vi "Dashboard Main.vi"() -> ()   [LabVIEW 2018]
uses:
  <vilib>/Utility/miscctls.llb/LVRowAndColumnTypeDef.ctl
  <vilib>/event_ctls.llb/eventvkey.ctl
  <vilib>/Rock Robotics/Network Tables/NT Read Numeric Array.vi
  <vilib>/Rock Robotics/WPI/Dashboard/WPI_DashboardLogging Global.vi
  <vilib>/vision/NI_Vision_Development_Module.lvlib
panel:
  in  "Camera Settings Right":T1={"Frame Rate"=30, "Compression"=30, "Size"=1, "DB Camera Config"=FALSE} {"Frame Rate" scale=1.0..30.0; "Compression" scale=100.0..-1.0; "Size" items=["640x480", "320x240", "160x120"]}
  in  "Camera Name Right":string(combo)="No Camera Selection"
  out "Camera Perf":string
  in  "Camera Settings":T1={"Frame Rate"=30, "Compression"=30, "Size"=1, "DB Camera Config"=FALSE} {"Frame Rate" scale=1.0..30.0; "Compression" scale=100.0..-1.0; "Size" items=["640x480", "320x240", "160x120"]}
  in  "TCP":refnum<k5>
  in  "Rec Mode":enum32{"Stop", "Record", "Playback"}(radio)
  out "Robot IP":string
  out "Image Message":string="Timeout in Camera Communications"
  in  "Dashboard Tab":T2(tab)
  in  "Select Auto":string(combo)="Select Autonomous ..."
  out "NT Connection":bool
  out "MotorChart R":cluster{"Numeric":dbl, "Numeric":dbl}(graph)
  out "MotorChart L":cluster{"Numeric":dbl, "Numeric":dbl}(graph)
  out "MotorSliders R":cluster{"MotorSlide1":dbl, "MotorSlide2":dbl} {"MotorSlide2" scale=-1.0..1.0 scale format="%#_2e"; "MotorSlide1" scale=-1.0..1.0 scale format="%#_2e"}
  out "MotorSliders L":cluster{"MotorSlide1":dbl, "MotorSlide2":dbl} {"MotorSlide2" scale=-1.0..1.0 scale format="%#_2e"; "MotorSlide1" scale=-1.0..1.0 scale format="%#_2e"}
  out "Gyro":dbl(knob) scale=0.0..360.0
  out "JS1 Z":dbl(slide) scale=-1.0..1.0 scale format="%#_2e"
  out "JS1 Graph":cluster{"X":dbl, "Y":dbl}[](graph)
  out "JS1 Buttons":T3
  out "JS2 Z":dbl(slide) scale=-1.0..1.0 scale format="%#_2e"
  out "JS2 Graph":cluster{"X":dbl, "Y":dbl}[](graph)
  out "JS2 Buttons":T3
  out "Mode":T4(ring)=enum."Auto Disabled"
  out "Right Camera Perf":cluster{"Bandwidth (Mbps)":dbl, "FPS":dbl}
  out "Camera Image Right":T5(plugin-control)
  in  "DB/String 9":string
  in  "DB/String 8":string
  in  "DB/String 7":string
  in  "DB/String 6":string
  in  "DB/String 5":string
  in  "DB/String 4":string
  in  "DB/String 3":string
  in  "DB/String 2":string
  in  "DB/String 1":string
  in  "DB/String 0":string
  in  "DB/Slider 0":dbl(slide) scale=0.0..5.0
  in  "DB/Slider 1":dbl(slide) scale=0.0..5.0
  in  "DB/Slider 2":dbl(slide) scale=0.0..5.0
  in  "DB/Slider 3":dbl(slide) scale=0.0..5.0
  out "DB/LED 3":bool
  out "DB/LED 2":bool
  out "DB/LED 1":bool
  out "DB/LED 0":bool
  in  "DB/Button 3":bool
  in  "DB/Button 2":bool
  in  "DB/Button 1":bool
  in  "DB/Button 0":bool caption="New Name"
  in  "Test Slider":dbl(slide) scale=0.0..100.0 scale format="%#_3g"
  in  "On/Off":bool caption="Solenoid"
  in  "Test Name":u16(ring) items=["Select the test to run..."]
  in  "Test Tree":string(tree)
  in  "Motor":cluster{"Value":dbl, "Enable":bool} {"Value" scale=-1.0..1.0 scale format="%#_3g"}
  out "Progress":T6 {"Test Progress" scale=0.0..100.0}
  in  "Rev/Fwd":cluster{"Forward":bool, "Reverse":bool}
  in  "Test Ring":u16(ring) items=["Monochrome", "Color"]
  out "Cmd Status":string
  in  "Execute Command":bool
  in  "Command Params":string[][](table)
  in  "Command Selection":i32(listbox)
  in  "CheckList":i32(listbox)
  out "Tree":string(tree)
  out "Camera Image":T5(plugin-control)
  out "Background":bool
  in  "Camera Name":string(combo)="No Camera Selection"
  # "HW"
  # "HW"
  # "Joysticks"
  # "Drive Motors"
  # "Front"
  # "Right"
  # "Left"
  # "Back"
  # "This tab is a great place for autonomous settings and robot-specific values.\nPlace controls and indicators inside this tab and match name to\nDashboard Variables on robot. You can also delete this comment."
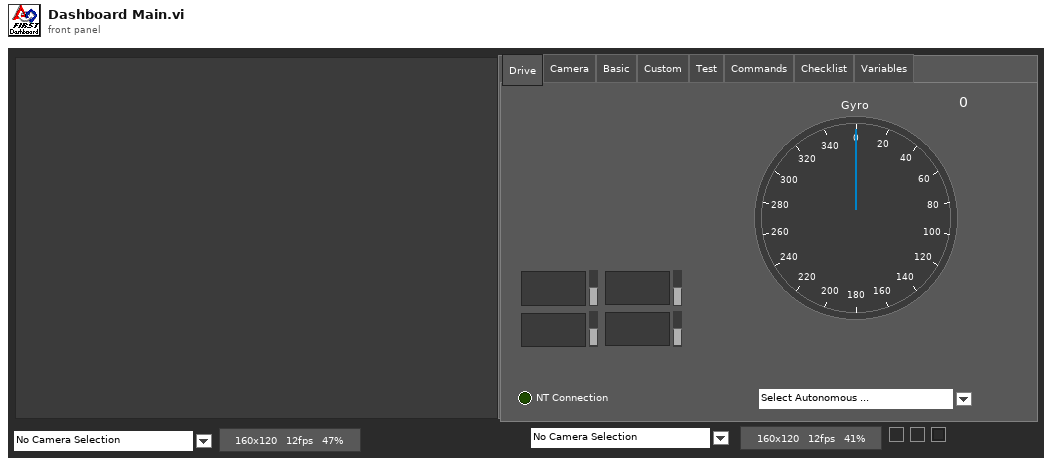
[diagram p1: front panel]
types:
  T1 = cluster{"Frame Rate":i32, "Compression":i32, "Size":u16, "DB Camera Config":bool}
  T2 = enum32{"Drive", "Camera", "Basic", "Custom", "Test", "Commands", "Checklist", "Variables"}
  T3 = cluster{bool, bool, bool, bool, bool, bool, bool, bool, bool, bool, bool, bool}
  T4 = enum8{"Tele-Op Disabled", "Tele-Op Enabled", "Auto Disabled", "Auto Enabled", "Test Disabled", "Test Enabled", "Disconnected", "No Code", "E-Stop"}
  T5 = typedef "IMAQ Image.ctl" = refnum<image>
  T6 = cluster{"Test Progress":u8, "Test Progress Text":string}
  T7 = typedef "Image Type" = u32
  T8 = cluster{"Save Path":path, "Interval (s)":dbl, "Keep":i32}
  T9 = cluster{"IDs":cluster{"RPC field ID":u16, "Unique ID":u16}, "String":string}
  T10 = cluster{"Error Strings":string, "Disable Counts":cluster{u16, u16}, "Rail Faults":cluster{u16, u16, u16}, "Robot IP":string, "DB Mode":u8, "Event Info":cluster{"Name":string, "Type":u8, "Number":u16, "Replay":u8}}
  T11 = cluster{"Storage":cluster{"Disk Free":u64, "RAM Block":u32, "RAM free":u32}, "CPU Utilization":cluster{"CPU % ISR":sgl, "CPU % Time Crit":sgl, "CPU % Timed Str":sgl, "CPU % High":sgl, "CPU % Above":sgl, "CPU % Normal":sgl, "CPU % Low":sgl}, "CAN":cluster{"% Bus Utilization":sgl, "Bus Off Cnt":u32, "TX_FIFO Full Cnt":u32, "Receive Error Cnt":u8, "Transmit Error Cnt":u8}, "HID":cluster{"HID Outputs":u32, "Rumble Low":u16, "Rumble High":u16}[]}
  T12 = cluster{"Status bits":cluster{"Test Mode":bool, "Autonomous":bool, "Enabled":bool, "Code Start":bool, "Brownout":bool, "Reserved 2":bool, "Reserved 3":bool, "E-Stop":bool}, "Code Trace":cluster{"Disabled":bool, "TeleOp":bool, "Auto":bool, "Test":bool}, "Controller Type":enum16{"unknown", "cRIO", "roboRio"}, "Code?":enum16{"unknown", "noCode", "code"}, "Battery V":dbl}
  T13 = cluster{"Control Bits":cluster{"TestMode":bool, "Autonomous":bool, "Enabled":bool, "FMS Present":bool, bool, bool, bool, "E-Stop":bool}, "Team Station ":u8, "Countdown":sgl, "Joystick Values":cluster{"Axes":dbl[], "Buttons":bool[], "POVs":i16[]}[]}
  T14 = cluster{"Axes":dbl[], "Buttons":bool[], "POVs":i16[]}[]
  T15 = cluster{"Axes":dbl[], "Buttons":bool[], "POVs":i16[]}
  T16 = cluster{"Buttons[0]":bool, "Buttons[1]":bool, "Buttons[2]":bool, "Buttons[3]":bool, "Buttons[4]":bool, "Buttons[5]":bool, "Buttons[6]":bool, "Buttons[7]":bool, "Buttons[8]":bool, "Buttons[9]":bool, "Buttons[10]":bool, "Buttons[11]":bool}
  T17 = cluster{"Camera Image":refnum<vi>, "Dashboard Tab":refnum<vi>, "Background":refnum<vi>, "Rec Mode":refnum<vi>, "Test Slider":refnum<vi>, "On/Off ":refnum<vi>, "Test Ring":refnum<vi>, "Rev/Fwd":refnum<vi>, "Test Name":refnum<vi>, "Motor":refnum<vi>, "Progress":refnum<vi>, "CheckList":refnum<vi>, "Tree":refnum<vi>, "Test Tree":refnum<vi>, "Command Params":refnum<vi>, "Command Selection":refnum<vi>, "Execute Command":refnum<vi>, "Cmd Status":refnum<vi>, "Camera Settings":refnum<vi>, "Camera Name":refnum<vi>, "Camera Perf":refnum<vi>, "Camera Settings Right":refnum<vi>, "Camera Name Right":refnum<vi>, "Camera Image Right":refnum<vi>}
  T18 = cluster{"Global Rectangle":i32[], "Contours":cluster{"Contour Type":u32, "ROI Type":u32, "Points":i32[]}[]}
  T19 = cluster{"Camera Name":string, string, "Saved DB Images Info":cluster{"Save Path":path, "Interval (s)":dbl, "Keep":i32}}
  T20 = cluster{"Camera Name Right":string, string, "Saved DB Images Info":cluster{"Save Path":path, "Interval (s)":dbl, "Keep":i32}}
  T21 = cluster{"Operation":enum16{"Update", "Clear"}, "Color Box":u32}[]
  T22 = typedef "eventvkey.ctl" = enum16{"ASCII", "Enter", "Return", "Shift", "Ctrl", "Alt", "Cmd", "Opt", "Caps", "NumLock", "Clear", "Break", "Up", "Down", "Left", "Right", "Insert", "Delete", "Home", "End", "PageUp", "PageDown", "Escape", "Help", "Pause", "ScrollLock", "F1", "F2", "F3", "F4", "F5", "F6", "F7", "F8", "F9", "F10", "F11", "F12", "F13", "F14", "F15", "F16", "F17", "F18", "F19", "F20", "F21", "F22", "F23", "F24", "Play", "VolumeUp", "VolumeDown", "Mute", "Two Byte Char"}
  T23 = cluster{"Image Size":bool, "Image Type":bool, "Pixel Value":bool, "ROI Information":bool, "Zoom Factor":bool}
  T24 = cluster{"Operation":enum16{"Update", "Clear"}, "Color Box":u32}
  T25 = typedef "LVRowAndColumnTypeDef.ctl" = cluster{"Row":i32, "Column":i32}
  T26 = cluster{"Shift":bool, "Ctrl":bool, "Alt":bool, "Cmd":bool, "Opt":bool}
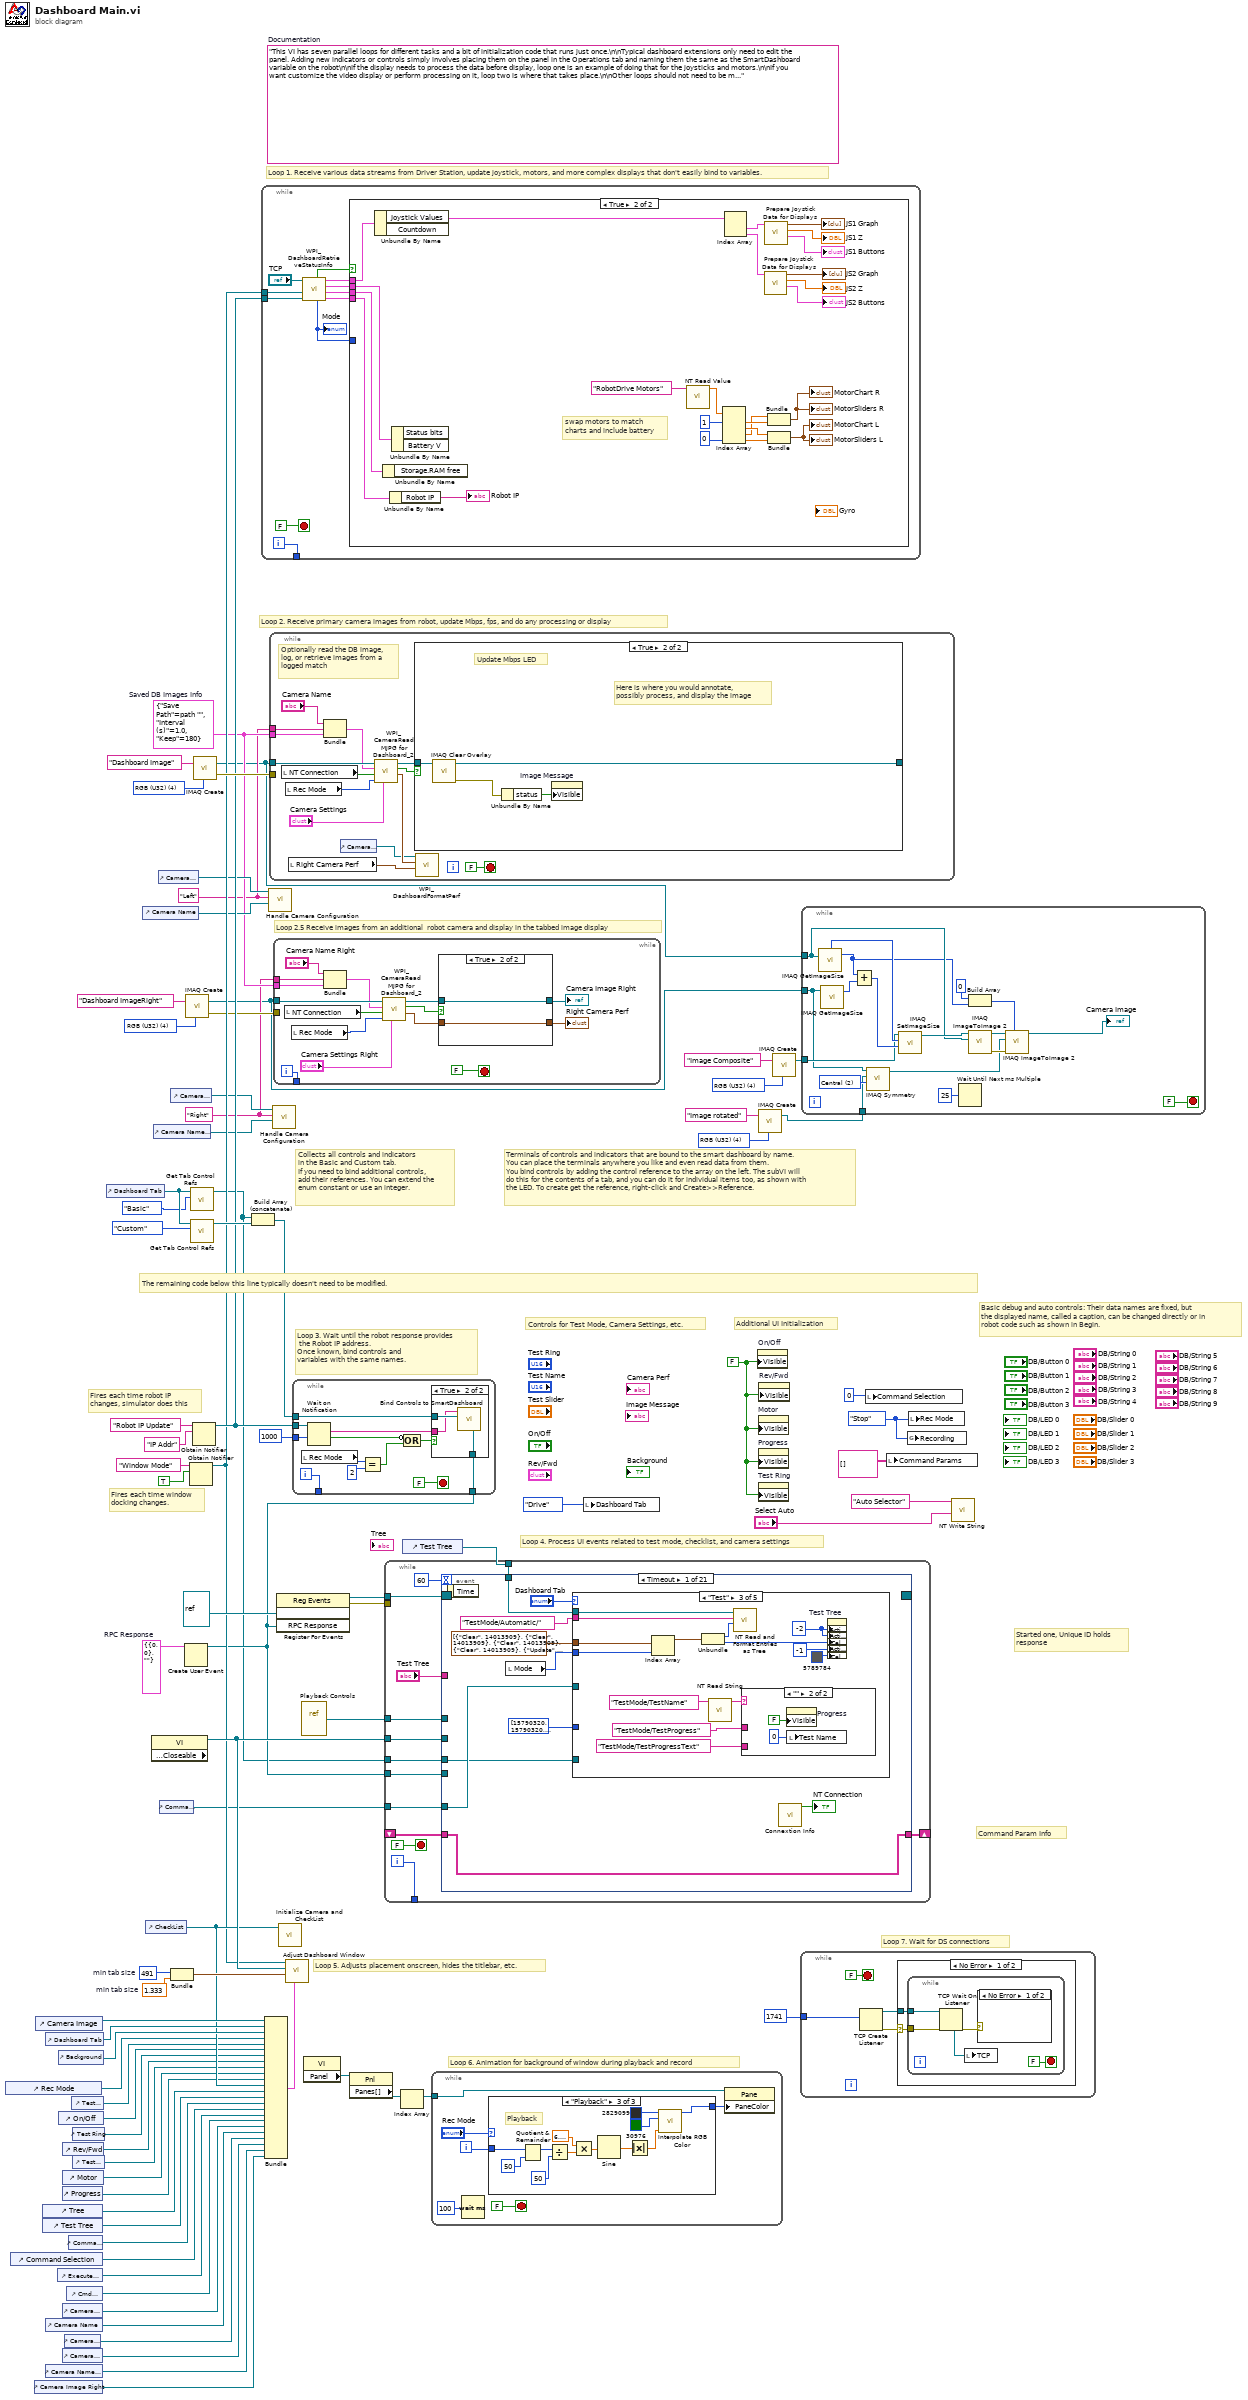
[diagram p0: block diagram]
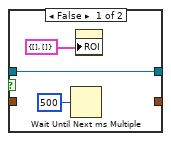
[diagram p2: hidden frame]
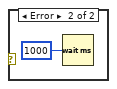
[diagram p3: hidden frame]
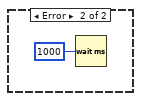
[diagram p4: hidden frame]
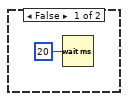
[diagram p5: hidden frame]
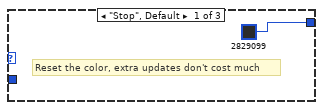
[diagram p6: hidden frame]
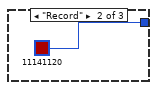
[diagram p7: hidden frame]
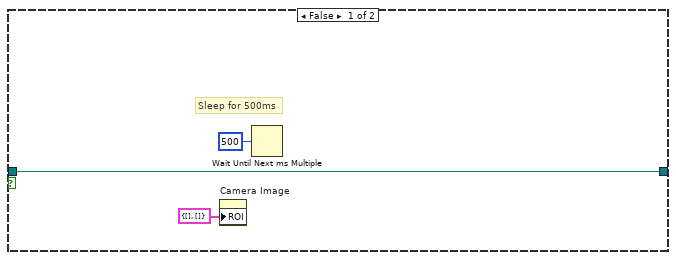
[diagram p9: hidden frame]
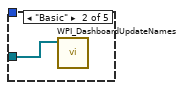
[diagram p11: hidden frame]
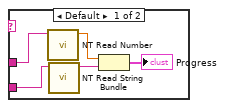
[diagram p12: hidden frame]
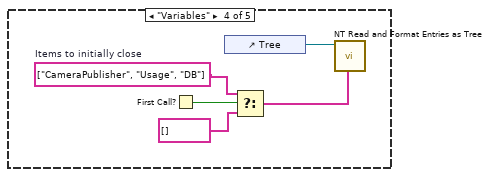
[diagram p13: hidden frame]
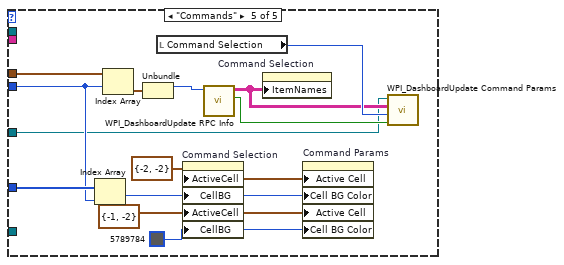
[diagram p14: hidden frame]
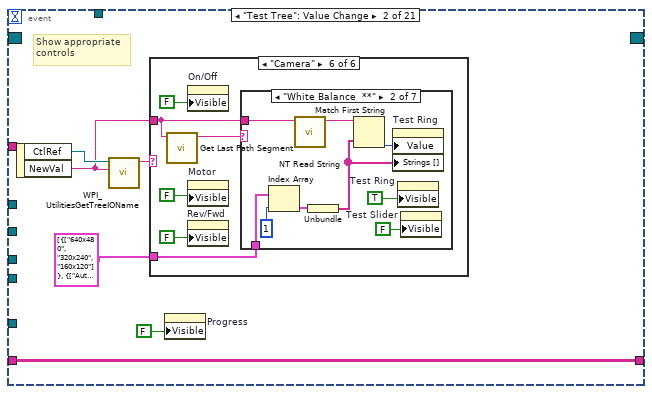
[diagram p15: hidden frame]
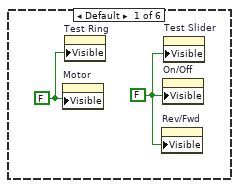
[diagram p16: hidden frame]
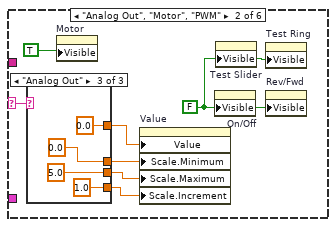
[diagram p17: hidden frame]
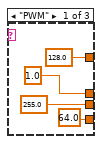
[diagram p18: hidden frame]
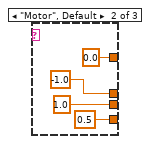
[diagram p19: hidden frame]
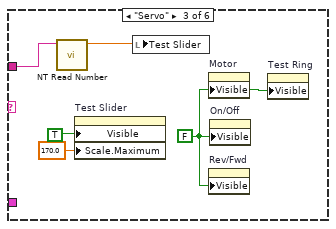
[diagram p20: hidden frame]
diagram:
  w2 = T7 4 items=["Grayscale (U8)", "Grayscale (I16)", "Grayscale (SGL)", "Complex (CSG)", "RGB (U32)", "HSL (U32)", "RGB (U64)"] ("Image Type")
  w8 = T7 4 items=["Grayscale (U8)", "Grayscale (I16)", "Grayscale (SGL)", "Complex (CSG)", "RGB (U32)", "HSL (U32)", "RGB (U64)"] ("Image Type")
  w11 = T8 {"Save Path"=path "", "Interval (s)"=1.0, "Keep"=180}  # Saved DB Images Info
  w10 = "Right"
  w9 = "Left"
  w20 = T7 4 items=["Grayscale (U8)", "Grayscale (I16)", "Grayscale (SGL)", "Complex (CSG)", "RGB (U32)", "HSL (U32)", "RGB (U64)"] ("Image Type")
  w36 = T9 {"IDs"={"RPC field ID"=0, "Unique ID"=0}, "String"=""}  # RPC Response
  w59 = 491  # min tab size
  w58 = 1.333  # min tab size
  w66 = enum32{"Stop", "Record", "Playback"}."Stop" ("Rec Mode")
  w43 = FALSE ("Visible")
  (unwired) "This VI has seven parallel loops for different tasks and a bit of initialization code that runs just once.\n\nTypical dashboard extensions only need to edit the panel. Adding new indicators or controls simply involves placing them on the panel in the Operations tab and naming them the same as the SmartDashboard variable on the robot\n\nIf the display needs to process the data before display, loop one is an example of doing that for the joysticks and motors.\n\nIf you want customize the video display or perform processing on it, loop two is where that takes place.\n\nOther loops should not need to be modified. They are pretty standard, and document the task they perform."  # Documentation
  w82 = T7 4 items=["Grayscale (U8)", "Grayscale (I16)", "Grayscale (SGL)", "Complex (CSG)", "RGB (U32)", "HSL (U32)", "RGB (U64)"] ("Image Type")
  # "Loop 2.5 Receive images from an additional  robot camera and display in the tabbed image display"
  # "Command Param Info"
  # "Started one, Unique ID holds\nresponse"
  # "Loop 7. Wait for DS connections"
  # "Basic debug and auto controls: Their data names are fixed, but\nthe displayed name, called a caption, can be changed directly or in\nrobot code such as shown in Begin."
  # "Controls for Test Mode, Camera Settings, etc."
  # "Additional UI Initialization"
  # "Loop 6. Animation for background of window during playback and record"
  # "Fires each time robot IP\nchanges, simulator does this"
  # "Fires each time window\ndocking changes."
  # "Collects all controls and indicators\nin the Basic and Custom tab.\nIf you need to bind additional controls,\nadd their references. You can extend the\nenum constant or use an integer."
  # "The remaining code below this line typically doesn't need to be modified."
  # "Loop 4. Process UI events related to test mode, checklist, and camera settings"
  # "Terminals of controls and indicators that are bound to the smart dashboard by name.\nYou can place the terminals anywhere you like and even read data from them.\nYou bind controls by adding the control reference to the array on the left. The subVI will\ndo this for the contents of a tab, and you can do it for individual items too, as shown with\nthe LED. To create get the reference, right-click and Create>>Reference."
  # "Loop 3. Wait until the robot response provides\n the Robot IP address.\nOnce known, bind controls and\nvariables with the same names."
  # "Loop 5. Adjusts placement onscreen, hides the titlebar, etc."
  # "Loop 1. Receive various data streams from Driver Station, update joystick, motors, and more complex displays that don't easily bind to variables."
  # "Loop 2. Receive primary camera images from robot, update Mbps, fps, and do any processing or display"
  n1 = control-ref of="Rec Mode"() -> (w49:refnum<vi>)
  n2 = control-ref of="Command Selection"() -> (w35:refnum<vi>)
  n3 = control-ref of="Camera Image Right"() -> (w14:refnum<vi>)
  n4 = control-ref of="Camera Image"() -> (w61:refnum<vi>)
  n5 = control-ref of="Tree"() -> (w53:refnum<vi>)
  n6 = control-ref of="Test Tree"() -> (w52:refnum<vi>)
  n7 = control-ref of="Dashboard Tab"() -> (w60:refnum<vi>)
  n8 = control-ref of="Camera Name"() -> (w26:refnum<vi>)
  n9 = control-ref of="Camera Name Right"() -> (w15:refnum<vi>)
  n10 = control-ref of="Execute Command"() -> (w37:refnum<vi>)
  n11 = control-ref of="Background"() -> (w56:refnum<vi>)
  n12 = control-ref of="On/Off"() -> (w47:refnum<vi>)
  n13 = control-ref of="Progress"() -> (w44:refnum<vi>)
  n14 = control-ref of="Camera Settings"() -> (w27:refnum<vi>)
  n15 = control-ref of="Camera Settings Right"() -> (w16:refnum<vi>)
  n16 = control-ref of="Rev/Fwd"() -> (w45:refnum<vi>)
  n17 = control-ref of="Motor"() -> (w50:refnum<vi>)
  n18 = control-ref of="Camera Perf"() -> (w25:refnum<vi>)
  n19 = control-ref of="Cmd Status"() -> (w31:refnum<vi>)
  n20 = control-ref of="Command Params"() -> (w38:refnum<vi>)
  n21 = control-ref of="Test Slider"() -> (w48:refnum<vi>)
  n22 = control-ref of="Test Ring"() -> (w46:refnum<vi>)
  n23 = control-ref of="Test Name"() -> (w51:refnum<vi>)
  n24 = control-ref of="Dashboard Tab"() -> (w64:refnum<vi>)
  n25 = control-ref of="Camera Name"() -> (w28:refnum<vi>)
  n26 = control-ref of="CheckList"() -> (w54:refnum<vi>)
  n27 = property class="VI" props=["Front Panel.Closeable"]() -> (reference out=w65:refnum<vi>)  [unwired: 2 in, 2 out]
  n28 = control-ref of="Camera Name Right"() -> (w17:refnum<vi>)
  n29 = control-ref of="Camera Settings"() -> (w29:refnum<vi>)
  n30 = control-ref of="Command Params"() -> (w30:refnum<vi>)
  n31 = control-ref of="Camera Settings Right"() -> (w18:refnum<vi>)
  n32 = Bundle("min tab size"=w59, "min tab size"=w58) -> (w57:cluster{"min tab size":i32, "min tab size":dbl})  [unwired: 1 in]
  n33 = Create User Event(user event datatype=w36) -> (user event=w32:refnum<user-event>)  [unwired: 1 in, 1 out]
  n34 = call "IMAQ Create"("Image Name"="Dashboard ImageRight", "Image Type"=w20) -> ("New Image"=w5:T5, "error out"=w19:errorcluster)  [unwired: 2 in, 1 out]
  n35 = Obtain Notifier(name (unnamed)="Window Mode", notification data type=TRUE) -> (notifier out=w41:refnum<notifier>)  [unwired: 2 in, 2 out]
  n36 = call <vilib>:"Get Tab Control Refs.vi"("Page Index"=T2."Basic" ("Dashboard Tab"), "TabControl in"=w64) -> ("ControlsOnPage"=w24:refnum<vi>[])  [unwired: 9 in]
  n37 = call <vilib>:"Get Tab Control Refs.vi"("Page Index"=T2."Custom" ("Dashboard Tab"), "TabControl in"=w64) -> ("ControlsOnPage"=w63:refnum<vi>[])  [unwired: 9 in]
  n38 = Obtain Notifier(name (unnamed)="Robot IP Update", notification data type="IP Addr" ("name (unnamed)")) -> (notifier out=w42:refnum<notifier>)  [unwired: 2 in, 2 out]
  n39 = call "IMAQ Create"("Image Name"="Dashboard Image", "Image Type"=w82) -> ("New Image"=w6:T5, "error out"=w80:errorcluster)  [unwired: 2 in, 1 out]
  n40 = Build Array (concatenate)(w24, w63) -> (w62:refnum<vi>[])
  n41 = while {
    tunnel: [w92] -> _
    tunnel: w42 -> [w86]
    tunnel: w41 -> [w83]
    i -> [w92]
    stop <- FALSE stop-if-true
    n42 = call <vilib>:"WPI_DashboardRetrieveStatusInfo.vi"("Binding Refnum"=w86, "Window Mode Notifier"=w83, "TCP Cnx"="TCP") -> ("Power and Errors"=w87:T10, "Robot Metrics"=w90:T11, "Status Info"=w91:T12, "Control Info"=w88:T13, "Robot Mode"=w85:T4, "Process?"=w89:bool)  [unwired: 3 in]
    "Mode" <- w85
    n43 = case shown="True" w89 {
      tunnel: w91 -> [_ w118]
      tunnel: w90 -> [_ w117]
      tunnel: w88 -> [_ w116]
      tunnel: w87 -> [_ w115]
      tunnel: w85 -> [_ _]
      frame False {
        n44 = Wait (ms)(milliseconds to wait=u32 20) -> ()  [unwired: 1 out]
      }
      frame True {
        # "swap motors to match\ncharts and include battery"
        n45 = Unbundle By Name(w116) -> ("Joystick Values"=w106:T14)  [unwired: 1 out]
        n46 = Unbundle By Name(w117) -> ()  [unwired: 1 out]
        n47 = Unbundle By Name(w115) -> ("Robot IP"=→"Robot IP":string)
        n48 = Unbundle By Name(w118) -> ()  [unwired: 2 out]
        n49 = call-poly <vilib>:"NT Read Value.vi"("Name"="RobotDrive Motors") -> ("Numeric Array"=w96:dbl[])  [unwired: 9 in, 1 out]
        n50 = Index Array(array=w96, index #1=1, index #4=0) -> (element #1=w110:dbl, element #2=w111:dbl, element #3=w109:dbl, element #4=w114:dbl)  [unwired: 2 in]
        n51 = Index Array(array=w106) -> (element #1=w105:T15, element #2=w101:T15)  [unwired: 2 in]
        n52 = call "Prepare Joystick Data for Displays.vi"("Joystick Values"=w101) -> ("Buttons"=→"JS2 Buttons":T16, "Z Axis"=→"JS2 Z":dbl, "Cartesian Data"=→"JS2 Graph":cluster{"X axis":dbl, "X axis":dbl}[])  [unwired: 8 in]
        n53 = call "Prepare Joystick Data for Displays.vi"("Joystick Values"=w105) -> ("Buttons"=→"JS1 Buttons":T16, "Z Axis"=→"JS1 Z":dbl, "Cartesian Data"=→"JS1 Graph":cluster{"X axis":dbl, "X axis":dbl}[])  [unwired: 8 in]
        n54 = Bundle("Numeric"=w109, "Numeric"=w110) -> (→"MotorChart R" →"MotorSliders R":cluster{"Numeric":dbl, "Numeric":dbl})  [unwired: 1 in]
        n55 = Bundle("Numeric"=w111, "Numeric"=w114) -> (→"MotorChart L" →"MotorSliders L":cluster{"Numeric":dbl, "Numeric":dbl})  [unwired: 1 in]
      }
    }
  }
  n56 = Bundle("Camera Image"=w61, "Dashboard Tab"=w60, "Background"=w56, "Rec Mode"=w49, "Test Slider"=w48, "On/Off"=w47, "Test Ring"=w46, "Rev/Fwd"=w45, "Test Name"=w51, "Motor"=w50, "Progress"=w44, "CheckList"=w54, "Tree"=w53, "Test Tree"=w52, "Command Params"=w38, "Command Selection"=w35, "Execute Command"=w37, "Cmd Status"=w31, "Camera Settings"=w27, "Camera Name"=w26, "Camera Perf"=w25, "Camera Settings Right"=w16, "Camera Name Right"=w15, "Camera Image Right"=w14) -> (w55:T17)  [unwired: 1 in]
  n57 = call "Handle Camera Configuration.vi"("CameraNameRef"=w28, "Display Name"=w9, "ClusterRef"=w29) -> ()  [unwired: 9 in]
  n58 = while {
    tunnel: w6 -> [w131]
    tunnel: w80 -> [_]
    tunnel: w11 -> [w125]
    tunnel: w9 -> [w122]
    stop <- FALSE stop-if-true
    # "Optionally read the DB image,\nlog, or retrieve images from a\nlogged match"
    n59 = local read "NT Connection"() -> (w126:bool)
    n60 = local read "Rec Mode"() -> (w128:enum32{"Stop", "Record", "Playback"})
    n61 = local read "Right Camera Perf"() -> (w120:cluster{"Bandwidth (Mbps)":dbl, "FPS":dbl})
    n62 = Bundle("Camera Name"="Camera Name", w122, "Saved DB Images Info"=w125) -> (w124:T19)  [unwired: 1 in]
    n63 = control-ref of="Camera Perf"() -> (w119:refnum<vi>)
    n64 = call <vilib>:"WPI_CameraRead MJPG for Dashboard_2.vi"("Camera Settings"="Camera Settings", "Rec Mode"=w128, "NT Connection"=w126, "Capture Info"=w124, "Image in"=w131) -> ("perf info"=w121:cluster{"Bandwidth (Mbps)":dbl, "fps":dbl}, "Active"=w129:bool, "Image\\ out"=w130:T5)  [unwired: 4 in]
    n65 = case shown="True" w129 {
      tunnel: w130 -> [w134 w137]
      tunnel: [w134 w136] -> _
      frame False {
        # "Sleep for 500ms"
        n66 = property on="Camera Image" class="ImageControl"("ROI"=T18 {"Global Rectangle"=[], "Contours"=[]}) -> ()  [unwired: 2 in, 2 out]
        n67 = Wait Until Next ms Multiple(millisecond multiple=u32 500) -> ()  [unwired: 1 out]
      }
      frame True {
        # "Here is where you would annotate,\npossibly process, and display the image"
        # "Update Mbps LED"
        n68 = call "IMAQ Clear Overlay"("Image"=w137) -> ("error out"=w138:errorcluster, "Image Out"=w136:T5)  [unwired: 2 in, 7 out]
        n69 = Unbundle By Name(w138) -> ("status"=w139:bool)
        n70 = property on="Image Message" class="Str"("Visible"=w139) -> ()  [unwired: 2 in, 2 out]
      }
    }
    n71 = call <vilib>:"WPI_DashboardFormatPerf.vi"("Right Camera Perf"=w120, "Performance"=w121, "String in"=w119) -> ()  [unwired: 9 in]
  }
  n72 = call "Handle Camera Configuration.vi"("CameraNameRef"=w17, "Display Name"=w10, "ClusterRef"=w18) -> ()  [unwired: 9 in]
  n73 = while {
    tunnel: w5 -> [w154]
    tunnel: w19 -> [_]
    tunnel: [w149] -> _
    tunnel: w11 -> [w145]
    tunnel: w10 -> [w142]
    i -> [w149]
    stop <- FALSE stop-if-true
    n74 = local read "NT Connection"() -> (w146:bool)
    n75 = local read "Rec Mode"() -> (w153:enum32{"Stop", "Record", "Playback"})
    n76 = Bundle("Camera Name Right"="Camera Name Right", w142, "Saved DB Images Info"=w145) -> (w144:T20)  [unwired: 1 in]
    n77 = call <vilib>:"WPI_CameraRead MJPG for Dashboard_2.vi"("Camera Settings"="Camera Settings Right", "Rec Mode"=w153, "NT Connection"=w146, "Capture Info"=w144, "Image in"=w154) -> ("perf info"=w140:cluster{"Bandwidth (Mbps)":dbl, "fps":dbl}, "Active"=w148:bool, "Image\\ out"=w151:T5)  [unwired: 4 in]
    n78 = case shown="True" w148 {
      tunnel: w151 -> [w156 w159]
      tunnel: [w156 w159] -> w147
      tunnel: [_ w158] -> w141
      tunnel: w140 -> [_ w158]
      frame False {
        n79 = Wait Until Next ms Multiple(millisecond multiple=u32 500) -> ()  [unwired: 1 out]
        n80 = property on="Camera Image Right" class="ImageControl"("ROI"=T18 {"Global Rectangle"=[], "Contours"=[]}) -> ()  [unwired: 2 in, 2 out]
      }
      frame True {
      }
    }
    "Camera Image Right" <- w147
    "Right Camera Perf" <- w141
  }
  n81 = register-events(refnum<vi> refnum, w32) -> (reference out=w70:refnum<event-registration>, error out=w69:errorcluster)  [unwired: 2 in]
  n82 = call "Initialize Camera and CheckList.vi"("ListBox in"=w54) -> ()  [unwired: 11 in]
  n83 = call "Adjust Dashboard Window.vi"("Sizing Refnums"=w55, "Size Constraints"=w57, "VI"=w65, "WIn Mode"=w41) -> ()  [unwired: 8 in]
  n84 = while {
    tunnel: w62 -> [w171]
    tunnel: w42 -> [w169]
    tunnel: [w167] -> _
    tunnel: u32 1000 ("milliseconds to wait") -> [w166]
    tunnel: w32 -> [w160]
    i -> [w167]
    stop <- FALSE stop-if-true
    n85 = local read "Rec Mode"() -> (w162:enum32{"Stop", "Record", "Playback"})
    n86 = Wait on Notification(notifier=w169, timeout in ms (-1)=w166) -> (notification=w168:string, timed out?=w164:bool)  [unwired: 2 in, 2 out]
    n87 = Equal?(x=w162, y=u16 2 ("Rec Mode")) -> (x = y?=w163:bool)
    n88 = Compound Arithmetic op=OR(invert w164, w163) -> (w165:bool)
    n89 = case shown="True" w165 {
      tunnel: w171 -> [_ w174]
      tunnel: w168 -> [_ w173]
      tunnel: w160 -> [_ w172]
      frame False {
      }
      frame True {
        n90 = call <vilib>:"Bind Controls to SmartDashboard.vi"("RPC ref"=w172, "Bound Control Refs"=w174, "Server IP Address"=w173) -> ()  [unwired: 9 in]
      }
    }
  }
  n91 = vi-ref "Playback Controls.vi"() -> (w71:refnum<vi>)
  n92 = property class="VI"() -> ("Panel"=w73:refnum<vi>)  [unwired: 2 in, 2 out]
  n93 = property class="Pnl"(reference=w73) -> ("Panes[]"=w74:refnum<vi>[])  [unwired: 1 in, 2 out]
  n94 = Index Array(array=w74) -> (element=w72:refnum<vi>)  [unwired: 1 in]
  n95 = control-ref of="Test Tree"() -> (w75:refnum<vi>)
  n96 = while {
    tunnel: [w184] -> _
    tunnel: w75 -> [w183]
    tunnel: w71 -> [w182]
    tunnel: w70 -> [w181]
    tunnel: w69 -> [_]
    tunnel: w65 -> [w180]
    tunnel: w32 -> [w179]
    tunnel: w30 -> [w178]
    shift-right: [w177] -> _
    shift-left: _ -> [w176]
    tunnel: w24 -> [w175]
    i -> [w184]
    stop <- FALSE stop-if-true
    n97 = event shown="[0] Timeout" {
      selector: w181 -> [_ _ _ _ _ _ _ _ _ _ _ _ _ _ _ _ _ _ _ _ _]
      dyn-events: [_ _ _ _ _ _ _ _ _ _ _ _ _ _ _ _ w444 _ _ _ _] -> _
      timeout: u32 60 ("milliseconds to wait") -> [_ _ _ _ _ _ _ _ _ _ _ _ _ _ _ _ _ _ _ _ _]
      tunnel: w183 -> [w196 _ _ _ _ _ _ _ _ _ _ _ _ _ _ _ _ _ _ _ _]
      tunnel: "Test Tree" -> [_ _ _ _ _ _ _ _ _ _ _ w411 w419 w421 w425 w433 _ _ _ _ _]
      tunnel: w182 -> [_ _ _ _ _ _ _ _ _ _ _ _ _ _ _ _ w446 _ w464 _ _]
      tunnel: w180 -> [_ _ _ _ _ _ _ _ _ _ _ _ _ _ _ _ w442 _ _ _ _]
      tunnel: w179 -> [_ _ _ _ _ _ _ _ _ _ _ _ _ _ _ _ w440 _ _ _ _]
      tunnel: w178 -> [w191 _ _ _ _ _ w362 _ _ _ _ _ _ _ _ _ _ _ _ _ _]
      tunnel: [w190 w239 w341 w346 w355 w359 w360 w369 w379 w386 w398 w410 w417 w420 w424 w432 w439 w459 w461 w465 w478] -> w177
      tunnel: w176 -> [w190 w239 w341 w346 w355 w359 w360 _ _ w386 w398 w410 w417 w420 w424 w432 w439 w459 w461 w465 w478]
      tunnel: w175 -> [w188 _ _ _ _ _ _ _ _ _ _ _ _ _ _ _ _ _ _ _ _]
      event Timeout {
        n98 = event-data() -> ()  [unwired: 1 in, 1 out]
        n99 = local read "Mode"() -> (w193:T4)
        n100 = case shown="\"Test\"" "Dashboard Tab" {
          tunnel: w196 -> [_ _ w212 _ _]
          tunnel: "TestMode/Automatic/" ("Name Pattern") -> [_ _ w211 _ _]
          tunnel: T21 [{"Operation"=enum."Clear", "Color Box"=14013909}, {"Operation"=enum."Clear", "Color Box"=14013909}, {"Operation"=enum."Clear", "Color Box"=14013909}, {"Operation"=enum."Clear", "Color Box"=14013909}, {"Operation"=enum."Update", "Color Box"=14013909}, {"Operation"=enum."Update", "Color Box"=16777215}, {"Operation"=enum."Clear", "Color Box"=14013909}, {"Operation"=enum."Clear", "Color Box"=14013909}, {"Operation"=enum."Clear", "Color Box"=14013909}] -> [_ _ w204 _ w232]
          tunnel: w193 -> [_ _ w203 _ w231]
          tunnel: u32[] [15790320, 15790320, 15790320, 15790320, 16777215, 16777215, 15790320, 15790320, 15790320] -> [_ _ _ _ w237]
          tunnel: w191 -> [_ _ _ _ w225]
          tunnel: w188 -> [_ w198 _ _ _]
          frame "Custom", Default {
          }
          frame "Basic" {
            n101 = call <vilib>:"WPI_DashboardUpdateNames.vi"("Controls on Tab"=w198) -> ()  [unwired: 11 in]
          }
          frame "Test" {
            w210 = -2 ("Active Item:Row Number")
            n102 = Index Array(array=w204, index=w203) -> (element=w205:T24)
            n103 = Unbundle(w205) -> ("Operation"=w206:enum16{"Update", "Clear"}, "Color Box"=w207:u32)
            n104 = call <vilib>:"NT Read String.vi"("Name"="TestMode/TestName") -> ("String"=w201:string)  [unwired: 9 in, 1 out]
            n105 = call <vilib>:"NT Read and Format Entries as Tree.vi"("Operation"=w206, "Name Pattern"=w211, "Tree Refnum"=w212) -> ()  [unwired: 7 in, 2 out]
            n106 = case shown="\"\"" w201 {
              tunnel: "TestMode/TestProgress" ("Name") -> [w214 _]
              tunnel: "TestMode/TestProgressText" ("Name") -> [w213 _]
              frame Default {
                n107 = call <vilib>:"NT Read Number.vi"("Name"=w214) -> ("Numeric"=w215:dbl)  [unwired: 9 in, 1 out]
                n108 = call <vilib>:"NT Read String.vi"("Name"=w213) -> ("String"=w216:string)  [unwired: 9 in, 1 out]
                n109 = Bundle("Numeric"=w215, "String"=w216) -> (→"Progress":cluster{"Numeric":dbl, "String":string})  [unwired: 1 in]
              }
              frame "" {
                n110 = property on="Progress" class="Clust (strict)"("Visible"=FALSE) -> ()  [unwired: 2 in, 2 out]
                n111 = local write "Test Name"(u16 0) -> ()
              }
            }
            n112 = property on="Test Tree" class="Tree (strict)"("Active Item Row Number"=w210, "ActiveColNum"=w210, "CellBG"=w207, "Active Item Row Number"=-1 ("Active Item:Row Number"), "CellBG"=u32 5789784 ("Color Box")) -> ()  [unwired: 2 in, 2 out]
          }
          frame "Variables" {
            w222 = string[] ["CameraPublisher", "Usage", "DB"]  # Items to initially close
            n113 = First Call?() -> (First Call?: T/F=w223:bool)
            n114 = control-ref of="Tree"() -> (w224:refnum<vi>)
            n115 = Select(t=w222, s=w223, f=string[] []) -> (s? t:f=w220:string[])
            n116 = call <vilib>:"NT Read and Format Entries as Tree.vi"("Tags to  Close"=w220, "Tree Refnum"=w224) -> ()  [unwired: 8 in, 2 out]
          }
          frame "Commands" {
            w233 = u32 5789784 ("Color Box")
            w234 = T25 {"Row"=-1, "Column"=-2} ("Active Cell:Active Cell")
            w236 = T25 {"Row"=-2, "Column"=-2} ("Active Cell:Active Cell")
            n117 = Index Array(array=w237, index=w231) -> (element=w235:u32)
            n118 = Index Array(array=w232, index=w231) -> (element=w230:T24)
            n119 = Unbundle(w230) -> ("Operation"=w229:enum16{"Update", "Clear"})  [unwired: 1 out]
            n120 = local read "Command Selection"() -> (w228:i32)
            n121 = property on="Command Selection" class="MCListbox (strict)"("ActiveCell"=w236, "CellBG"=w235, "ActiveCell"=w234, "CellBG"=w233) -> ()  [unwired: 2 in, 2 out]
            n122 = call <vilib>:"WPI_DashboardUpdate RPC Info.vi"("Operation"=w229) -> ("update"=w227:bool, "commands"=w226:string[][])  [unwired: 9 in]
            n123 = property on="Command Selection" class="MCListbox (strict)"("ItemNames"=w226) -> ()  [unwired: 2 in, 2 out]
            n124 = property on="Command Params" class="Tbl (strict)"("Active Cell"=w236, "Cell BG Color"=w235, "Active Cell"=w234, "Cell BG Color"=w233) -> ()  [unwired: 2 in, 2 out]
            n125 = call <vilib>:"WPI_DashboardUpdate Command Params.vi"("Update"=w227, "NewVal"=w228, "Commands"=w226, "Param Tbl"=w225) -> ()  [unwired: 7 in, 1 out]
          }
        }
        n126 = call <vilib>:"Connextion Info.vi"() -> ("Connected"=→"NT Connection":bool)  [unwired: 10 in, 1 out]
      }
      event "Test Tree": Value Change {
        # "Show appropriate\ncontrols"
        n127 = event-data() -> ("CtlRef"=w242:refnum<vi>, "NewVal"=w240:string)  [unwired: 1 in]
        n128 = call <vilib>:"WPI_UtilitiesGetTreeIOName.vi"("NewVal"=w240, "TreeControl in"=w242) -> ("I/O Name"=w243:string)  [unwired: 9 in]
        n129 = case shown="\"Camera\"" w243 {
          selector: w243 -> [_ w250 _ w272 w281 _]
          tunnel: w240 -> [_ _ w269 w271 _ w288]
          tunnel: cluster{string[]}[] [{["640x480", "320x240", "160x120"]}, {["Auto", "Fixed indoor", "Fixed outdoor 1", "Fixed outdoor 2", "Fixed fluorescent 1", "Fixed fluorescent 2", "Hold current"]}, {["Auto", "Flicker-free 50 Hz", "Flicker-free 60 Hz", "Hold current"]}, {["None", "Prioritize frame rate", "Prioritize image quality"]}, {["Monochrome", "Color"]}] -> [_ _ _ _ _ w287]
          frame Default {
            w245 = FALSE ("Visible")
            w244 = FALSE ("Visible")
            n130 = property on="Motor" class="Clust (strict)"("Visible"=w244) -> ()  [unwired: 2 in, 2 out]
            n131 = property on="Test Ring" class="Ring (strict)"("Visible"=w244) -> ()  [unwired: 2 in, 2 out]
            n132 = property on="Rev/Fwd" class="Clust (strict)"("Visible"=w245) -> ()  [unwired: 2 in, 2 out]
            n133 = property on="On/Off" class="Bool (strict)"("Visible"=w245) -> ()  [unwired: 2 in, 2 out]
            n134 = property on="Test Slider" class="Slide (strict)"("Visible"=w245) -> ()  [unwired: 2 in, 2 out]
          }
          frame "Analog Out", "Motor", "PWM" {
            w251 = FALSE ("Visible")
            n135 = case shown="\"Analog Out\"" w250 {
              tunnel: [1.0 ("Value") -1.0 ("Value") 0.0 ("Value")] -> w249
              tunnel: [255.0 ("Value") 1.0 ("Value") 5.0 ("Value")] -> w248
              tunnel: [128.0 ("Value") 0.0 ("Value") 0.0 ("Value")] -> w247
              tunnel: [64.0 ("Value") 0.5 ("Value") 1.0 ("Value")] -> w246
              frame "PWM" {
              }
              frame "Motor", Default {
              }
              frame "Analog Out" {
              }
            }
            n136 = property on="Motor" class="Clust (strict)"("Visible"=TRUE) -> ()  [unwired: 2 in, 2 out]
            n137 = property on="Value" class="Slide (strict)"("Value"=w247, "Scale.Minimum"=w249, "Scale.Maximum"=w248, "Scale.Increment"=w246) -> ()  [unwired: 2 in, 2 out]
            n138 = property on="On/Off" class="Bool (strict)"("Visible"=w251) -> ()  [unwired: 2 in, 2 out]
            n139 = property on="Test Slider" class="Slide (strict)"("Visible"=w251) -> ()  [unwired: 2 in, 2 out]
            n140 = property on="Test Ring" class="Ring (strict)"("Visible"=w251) -> ()  [unwired: 2 in, 2 out]
            n141 = property on="Rev/Fwd" class="Clust (strict)"("Visible"=w251) -> ()  [unwired: 2 in, 2 out]
          }
          frame "Servo" {
            w267 = FALSE ("Visible")
            n142 = call <vilib>:"NT Read Number.vi"("Name"=w269) -> ("Numeric"=w268:dbl)  [unwired: 9 in, 1 out]
            n143 = property on="Test Slider" class="Slide (strict)"("Visible"=TRUE, "Scale.Maximum"=170.0 ("Scale.Range:Maximum")) -> ()  [unwired: 2 in, 2 out]
            n144 = local write "Test Slider"(w268) -> ()
            n145 = property on="Motor" class="Clust (strict)"("Visible"=w267) -> ()  [unwired: 2 in, 2 out]
            n146 = property on="Rev/Fwd" class="Clust (strict)"("Visible"=w267) -> ()  [unwired: 2 in, 2 out]
            n147 = property on="On/Off" class="Bool (strict)"("Visible"=w267) -> ()  [unwired: 2 in, 2 out]
            n148 = property on="Test Ring" class="Ring (strict)"("Visible"=w267) -> ()  [unwired: 2 in, 2 out]
          }
          frame "Relay", "Solenoid" {
            w270 = FALSE ("Visible")
            n149 = property on="Motor" class="Clust (strict)"("Visible"=w270) -> ()  [unwired: 2 in, 2 out]
            n150 = property on="Test Slider" class="Slide (strict)"("Visible"=w270) -> ()  [unwired: 2 in, 2 out]
            n151 = Search and Replace String(input string=w271, search string="/Value  **", replace string="/Direction") -> (result string=w277:string)  [unwired: 5 in, 3 out]
            n152 = property on="Test Ring" class="Ring (strict)"("Visible"=w270) -> ()  [unwired: 2 in, 2 out]
            n153 = call <vilib>:"NT Read String.vi"("Name"=w277) -> ("String"=w275:string)  [unwired: 9 in, 1 out]
            n154 = Equal?(x="Both directions", y=w275) -> (x = y?=w273:bool)
            n155 = Not(x=w273) -> (.not. x?=w274:bool)
            n156 = property on="Rev/Fwd" class="Clust (strict)"("Visible"=w273) -> ()  [unwired: 2 in, 2 out]
            n157 = property on="On/Off" class="Bool (strict)"("Visible"=w274, "Caption.Text"=w272) -> ()  [unwired: 2 in, 2 out]
          }
          frame "Compressor", "Digital Out" {
            w280 = FALSE ("Visible")
            # "Get direction and finish"
            n158 = property on="Motor" class="Clust (strict)"("Visible"=w280) -> ()  [unwired: 2 in, 2 out]
            n159 = property on="Test Slider" class="Slide (strict)"("Visible"=w280) -> ()  [unwired: 2 in, 2 out]
            n160 = property on="Test Ring" class="Ring (strict)"("Visible"=w280) -> ()  [unwired: 2 in, 2 out]
            n161 = property on="On/Off" class="Bool (strict)"("Visible"=TRUE, "Caption.Text"=w281) -> ()  [unwired: 2 in, 2 out]
            n162 = property on="Rev/Fwd" class="Clust (strict)"("Visible"=FALSE) -> ()  [unwired: 2 in, 2 out]
          }
          frame "Camera" {
            n163 = call <vilib>:"Get Last Path Segment.vi"("String in"=w288) -> ("String out"=w289:string)  [unwired: 10 in]
            n164 = property on="On/Off" class="Bool (strict)"("Visible"=FALSE) -> ()  [unwired: 2 in, 2 out]
            n165 = property on="Motor" class="Clust (strict)"("Visible"=FALSE) -> ()  [unwired: 2 in, 2 out]
            n166 = property on="Rev/Fwd" class="Clust (strict)"("Visible"=FALSE) -> ()  [unwired: 2 in, 2 out]
            n167 = case shown="\"White Balance  **\"" w289 {
              tunnel: w288 -> [w295 w304 w313 w322 w331 _ w337]
              tunnel: w287 -> [w293 w301 w310 w319 w328 _ _]
              frame "Size  **" {
                n168 = Index Array(array=w293) -> (element=w292:cluster{string[]})  [unwired: 1 in]
                n169 = call <vilib>:"NT Read String.vi"("Name"=w295) -> ("String"=w294:string)  [unwired: 9 in, 1 out]
                n170 = Unbundle(w292) -> (w290:string[])
                n171 = Match First String(2:w290, 3:w294) -> (0:w291:i32)  [unwired: 1 out]
                n172 = property on="Test Ring" class="Ring (strict)"("Value"=w291, "Strings []"=w290) -> ()  [unwired: 2 in, 2 out]
                n173 = property on="Test Ring" class="Ring (strict)"("Visible"=TRUE) -> ()  [unwired: 2 in, 2 out]
                n174 = property on="Test Slider" class="Slide (strict)"("Visible"=FALSE) -> ()  [unwired: 2 in, 2 out]
              }
              frame "White Balance  **" {
                n175 = Index Array(array=w301, index=1) -> (element=w302:cluster{string[]})
                n176 = call <vilib>:"NT Read String.vi"("Name"=w304) -> ("String"=w303:string)  [unwired: 9 in, 1 out]
                n177 = Unbundle(w302) -> (w299:string[])
                n178 = Match First String(2:w299, 3:w303) -> (0:w298:i32)  [unwired: 1 out]
                n179 = property on="Test Ring" class="Ring (strict)"("Value"=w298, "Strings []"=w299) -> ()  [unwired: 2 in, 2 out]
                n180 = property on="Test Ring" class="Ring (strict)"("Visible"=TRUE) -> ()  [unwired: 2 in, 2 out]
                n181 = property on="Test Slider" class="Slide (strict)"("Visible"=FALSE) -> ()  [unwired: 2 in, 2 out]
              }
              frame "Exposure  **" {
                n182 = Index Array(array=w310, index=2) -> (element=w311:cluster{string[]})
                n183 = call <vilib>:"NT Read String.vi"("Name"=w313) -> ("String"=w312:string)  [unwired: 9 in, 1 out]
                n184 = Unbundle(w311) -> (w307:string[])
                n185 = Match First String(2:w307, 3:w312) -> (0:w308:i32)  [unwired: 1 out]
                n186 = property on="Test Ring" class="Ring (strict)"("Value"=w308, "Strings []"=w307) -> ()  [unwired: 2 in, 2 out]
                n187 = property on="Test Ring" class="Ring (strict)"("Visible"=TRUE) -> ()  [unwired: 2 in, 2 out]
                n188 = property on="Test Slider" class="Slide (strict)"("Visible"=FALSE) -> ()  [unwired: 2 in, 2 out]
              }
              frame "Exposure Priority  **" {
                n189 = Index Array(array=w319, index=3) -> (element=w320:cluster{string[]})
                n190 = call <vilib>:"NT Read String.vi"("Name"=w322) -> ("String"=w321:string)  [unwired: 9 in, 1 out]
                n191 = Unbundle(w320) -> (w316:string[])
                n192 = Match First String(2:w316, 3:w321) -> (0:w317:i32)  [unwired: 1 out]
                n193 = property on="Test Ring" class="Ring (strict)"("Value"=w317, "Strings []"=w316) -> ()  [unwired: 2 in, 2 out]
                n194 = property on="Test Ring" class="Ring (strict)"("Visible"=TRUE) -> ()  [unwired: 2 in, 2 out]
                n195 = property on="Test Slider" class="Slide (strict)"("Visible"=FALSE) -> ()  [unwired: 2 in, 2 out]
              }
              frame "Color Enable  **" {
                n196 = Index Array(array=w328, index=4) -> (element=w329:cluster{string[]})
                n197 = call <vilib>:"NT Read String.vi"("Name"=w331) -> ("String"=w330:string)  [unwired: 9 in, 1 out]
                n198 = Unbundle(w329) -> (w325:string[])
                n199 = Match First String(2:w325, 3:w330) -> (0:w326:i32)  [unwired: 1 out]
                n200 = property on="Test Ring" class="Ring (strict)"("Value"=w326, "Strings []"=w325) -> ()  [unwired: 2 in, 2 out]
                n201 = property on="Test Ring" class="Ring (strict)"("Visible"=TRUE) -> ()  [unwired: 2 in, 2 out]
                n202 = property on="Test Slider" class="Slide (strict)"("Visible"=FALSE) -> ()  [unwired: 2 in, 2 out]
              }
              frame Default {
                n203 = property on="Test Ring" class="Ring (strict)"("Visible"=FALSE) -> ()  [unwired: 2 in, 2 out]
                n204 = property on="Test Slider" class="Slide (strict)"("Visible"=FALSE) -> ()  [unwired: 2 in, 2 out]
              }
              frame "Brightness  **", "Color Level  **", "Compression  **", "FPS  **", "Sharpness  **" {
                n205 = call <vilib>:"NT Read Number.vi"("Name"=w337) -> ("Numeric"=w336:dbl)  [unwired: 9 in, 1 out]
                n206 = local write "Test Slider"(w336) -> ()
                n207 = property on="Test Slider" class="Slide (strict)"("Visible"=TRUE, "Scale.Maximum"=100.0 ("Scale.Range:Maximum")) -> ()  [unwired: 2 in, 2 out]
                n208 = property on="Test Ring" class="Ring (strict)"("Visible"=FALSE) -> ()  [unwired: 2 in, 2 out]
              }
            }
          }
        }
        n209 = property on="Progress" class="Clust (strict)"("Visible"=FALSE) -> ()  [unwired: 2 in, 2 out]
      }
      event "Test Name": Mouse Enter {
        # "Populate the ring with the list of tests"
        n210 = event-data() -> ()  [unwired: 1 in, 1 out]
        n211 = call <vilib>:"NT Read String Array.vi"("Name"="TestMode/TestList") -> ("String Array"=w345:string[])  [unwired: 9 in, 1 out]
        n212 = Build Array (concatenate)("Select the test to run...", w345) -> (w344:string[])
        n213 = property on="Test Name" class="Ring (strict)"("Strings []"=w344) -> ()  [unwired: 2 in, 2 out]
      }
      event "Test Name": Value Change {
        w347 = FALSE ("Visible")
        # "Tell the robot the test name to run"
        n214 = event-data() -> ("NewVal"=w351:u16)  [unwired: 1 in]
        n215 = property on="Test Name" class="Ring (strict)"() -> ("Strings []"=w352:string[])  [unwired: 2 in, 2 out]
        n216 = local write "Progress"(T6 {"Test Progress"=0, "Test Progress Text"=""} ("Progress")) -> ()
        n217 = Index Array(array=w352, index=w351) -> (element=w350:string)
        n218 = call <vilib>:"NT Write String.vi"("String"=w350, "Name"="TestMode/TestName") -> ()  [unwired: 9 in, 1 out]
        n219 = property on="Progress" class="Clust (strict)"("Visible"=TRUE) -> ()  [unwired: 2 in, 2 out]
        n220 = property on="Motor" class="Clust (strict)"("Visible"=w347) -> ()  [unwired: 2 in, 2 out]
        n221 = property on="Test Slider" class="Slide (strict)"("Visible"=w347) -> ()  [unwired: 2 in, 2 out]
        n222 = property on="On/Off" class="Bool (strict)"("Visible"=w347) -> ()  [unwired: 2 in, 2 out]
        n223 = property on="Rev/Fwd" class="Clust (strict)"("Visible"=w347) -> ()  [unwired: 2 in, 2 out]
        n224 = property on="Test Ring" class="Ring (strict)"("Visible"=w347) -> ()  [unwired: 2 in, 2 out]
      }
      event "Select Auto": Mouse Enter {
        # "Populate the combo box with the list of autonomous options"
        n225 = event-data() -> ()  [unwired: 1 in, 1 out]
        n226 = call <vilib>:"NT Read String Array.vi"("Name"="Auto List") -> ("String Array"=w354:string[])  [unwired: 9 in, 1 out]
        n227 = property on="Select Auto" class="CmbBox"("Strings[]"=w354) -> ()  [unwired: 2 in, 2 out]
      }
      event "Select Auto": Value Change {
        # "User modified the Auto Selection. Write to NT variable so robot knows."
        n228 = event-data() -> ("NewVal"=w357:string)  [unwired: 1 in]
        n229 = call <vilib>:"NT Write String.vi"("String"=w357, "Name"="Auto Selector") -> ()  [unwired: 9 in, 1 out]
      }
      event "Command Selection": Value Change {
        # "Get the params and show in table"
        n230 = event-data() -> ("NewVal"=w363:i32)  [unwired: 1 in]
        n231 = property on="Command Selection" class="MCListbox (strict)"() -> ("ItemNames"=w361:string[][])  [unwired: 2 in, 2 out]
        n232 = call <vilib>:"WPI_DashboardUpdate Command Params.vi"("NewVal"=w363, "Commands"=w361, "Param Tbl"=w362) -> ()  [unwired: 8 in, 1 out]
      }
      event "Execute Command": Value Change {
        # "Started one, Unique ID holds\nresponse"
        n233 = event-data() -> ()  [unwired: 1 in, 1 out]
        n234 = property on="Command Selection" class="MCListbox (strict)"() -> ("ItemNames"=w374:string[][])  [unwired: 2 in, 2 out]
        n235 = Index Array(array=w374, index (row)="Command Selection", index (col)=0) -> (element=w372:string)
        n236 = call <vilib>:"Invoke Commands.vi"("Command Params"="Command Params", "Function Name"=w372) -> ("Params"=w368:u8, "Started"=w367:bool)  [unwired: 7 in, 1 out]
        n237 = Array Subset(array="Command Params", length (row)=w368) -> (w369:string[][])  [unwired: 3 in]
        n238 = Select(t="Executing" ("Cmd Status"), s=w367, f="" ("Cmd Status")) -> (s? t:f=→"Cmd Status":string)
      }
      event "Command Selection": Double Click {
        n239 = event-data() -> ("Row"=w382:i32)  [unwired: 1 in]
        n240 = property on="Command Selection" class="MCListbox (strict)"() -> ("ItemNames"=w385:string[][])  [unwired: 2 in, 2 out]
        n241 = local read "Command Params"() -> (w381:string[][])
        n242 = Index Array(array=w385, index (row)=w382, index (col)=0) -> (element=w383:string)
        n243 = call <vilib>:"Invoke Commands.vi"("Command Params"=w381, "Function Name"=w383) -> ("Params"=w380:u8, "Started"=w375:bool)  [unwired: 7 in, 1 out]
        n244 = Array Subset(array=w381, length (row)=w380) -> (w379:string[][])  [unwired: 3 in]
        n245 = Select(t="Executing" ("Cmd Status"), s=w375, f="" ("Cmd Status")) -> (s? t:f=w376:string)
        n246 = local write "Cmd Status"(w376) -> ()
      }
      event "CheckList": Double Click {
        # "Shift clears all"
        # "Update symbols on the listbox"
        n247 = event-data() -> ("PlatMods.Shift"=w387:bool, "Row"=w389:i32)  [unwired: 1 in]
        n248 = case shown="True" w387 {
          tunnel: w389 -> [w393 _]
          tunnel: 1 -> [w392 _]
          frame False {
            n249 = property on="CheckList" class="LstBox (strict)"() -> ("Item Symbols"=w391:i32[])  [unwired: 2 in, 2 out]
            n250 = Replace Array Subset(array=w391, new element=w392, index=w393) -> (w390:i32[])
            n251 = property on="CheckList" class="LstBox (strict)"("Item Symbols"=w390) -> ()  [unwired: 2 in, 2 out]
          }
          frame True {
            w394 = 0 ("Top Row")
            n252 = property on="CheckList" class="LstBox (strict)"() -> ("Number of Rows"=w396:u32)  [unwired: 2 in, 2 out]
            n253 = Initialize Array(0, w396) -> (w395:i32[])
            n254 = property on="CheckList" class="LstBox (strict)"("Top Row"=w394, "Value"=w394, "Item Symbols"=w395) -> ()  [unwired: 2 in, 2 out]
          }
        }
      }
      event "CheckList": Key Down {
        # "Update symbols on the listbox\nLeft and right keys check and uncheck"
        n255 = event-data() -> ("VKey"=w400:T22)  [unwired: 1 in]
        n256 = case shown="\"Left\", \"Right\"" w400 {
          selector: w400 -> [w405 _]
          tunnel: eventvkey."Left" ("VKey") -> [w403 _]
          frame "Left", "Right" {
            n257 = Equal?(x=w403, y=w405) -> (x = y?=w404:bool)
            n258 = Select(t=0, s=w404, f=1) -> (s? t:f=w406:i32)
            n259 = property on="CheckList" class="LstBox (strict)"() -> ("Item Symbols"=w409:i32[])  [unwired: 2 in, 2 out]
            n260 = Replace Array Subset(array=w409, new element=w406, index="CheckList") -> (w408:i32[])
            n261 = property on="CheckList" class="LstBox (strict)"("Item Symbols"=w408) -> ()  [unwired: 2 in, 2 out]
          }
          frame Default {
          }
        }
      }
      event "Motor.Enable": Value Change {
        # "When the test mode otor enable helper is set, update that\ntree row item's value"
        n262 = event-data() -> ("NewVal"=w415:bool)  [unwired: 1 in]
        n263 = Unbundle("Motor") -> ("Value"=w414:dbl)  [unwired: 1 out]
        n264 = Select(t=w414, s=w415, f=0.0) -> (s? t:f=w412:dbl)
        n265 = call <vilib>:"NT Write Number.vi"("Numeric"=w412, "Name"=w411) -> ()  [unwired: 9 in, 1 out]
      }
      event "Test Slider": Value Change {
        # "When the test mode slider helper is set, update that\ntree row item's value"
        n266 = event-data() -> ("NewVal"=w418:dbl)  [unwired: 1 in]
        n267 = call <vilib>:"NT Write Number.vi"("Numeric"=w418, "Name"=w419) -> ()  [unwired: 9 in, 1 out]
      }
      event "On/Off": Value Change {
        # "When the test mode on/off helper value is set, update that\ntree row item's value"
        n268 = event-data() -> ("NewVal"=w423:bool)  [unwired: 1 in]
        n269 = Boolean To (0,1)(Boolean=w423) -> (0, 1=w422:i16)
        n270 = call <vilib>:"NT Write Number.vi"("Numeric"=w422, "Name"=w421) -> ()  [unwired: 9 in, 1 out]
      }
      event "Rev/Fwd": Value Change {
        # "When the test mode helper value for relays is set, update that\ntree row item's value"
        n271 = event-data() -> ("NewVal.Forward"=w431:bool, "NewVal.Reverse"=w430:bool)  [unwired: 1 in]
        n272 = Boolean To (0,1)(Boolean=w431) -> (0, 1=w427:i16)
        n273 = Boolean To (0,1)(Boolean=w430) -> (0, 1=w429:i16)
        n274 = Negate(x=w429) -> (-x=w428:i16)
        n275 = Add(x=w427, y=w428) -> (x+y=w426:i16)
        n276 = call <vilib>:"NT Write Number.vi"("Numeric"=w426, "Name"=w425) -> ()  [unwired: 9 in, 1 out]
      }
      event "Test Ring": Value Change {
        # "When a test mode helper value is selected from the ring,\nset the tree item's variable to the string value"
        n277 = event-data() -> ("NewVal"=w435:u16)  [unwired: 1 in]
        n278 = property on="Test Ring" class="Ring (strict)"() -> ("Strings []"=w436:string[])  [unwired: 2 in, 2 out]
        n279 = Index Array(array=w436, index=w435) -> (element=w434:string)
        n280 = call <vilib>:"NT Write String.vi"("String"=w434, "Name"=w433) -> ()  [unwired: 9 in, 1 out]
      }
      event "Rec Mode": Value Change {
        # "Update globals for recording mode and path to read log from.\nClear when logging and let NetworkTables set path for vision to\nuse."
        n281 = event-data() -> ("NewVal"=w447:enum32{"Stop", "Record", "Playback"})  [unwired: 1 in]
        n282 = global write "WPI_DashboardLogging Global.vi" "Logging Filename"(path "") -> ()
        n283 = global write "WPI_DashboardLogging Global.vi" "Recording"(w447) -> ()
        n284 = case shown="\"Playback\"" w447 {
          tunnel: w446 -> [_ w449 w458]
          tunnel: [_ _ w457] -> w444
          tunnel: [_ _ w456] -> _
          tunnel: w442 -> [_ _ w454]
          tunnel: cluster{i32, i32} {-250, 170} -> [_ _ w453]
          tunnel: [_ _ T23 {"Image Size"=TRUE, "Image Type"=TRUE, "Pixel Value"=TRUE, "ROI Information"=TRUE, "Zoom Factor"=FALSE} ("Image Information Shown:All Elements")] -> w437
          tunnel: [_ _ TRUE ("Zoom Factor")] -> w438
          tunnel: w440 -> [_ _ w450]
          frame Default {
          }
          frame "Stop", "Record" {
            # "Place Window too"
            n285 = invoke class="VI" method="FP.Close"(reference=w449) -> (reference out=w448:refnum<vi>)  [unwired: 2 in, 2 out]
            n286 = invoke class="VI" method="Abort VI"(reference=w448) -> ()  [unwired: 2 in, 3 out]
          }
          frame "Playback" {
            n287 = call "Open Playback Panel.vi"("Offset"=w453, "DB VI Ref"=w454, "Playback in"=w458) -> ("Playback out"=w455:refnum<vi>)  [unwired: 8 in]
            n288 = register-events(w455, w450) -> (reference out=w457:refnum<event-registration>, error out=w456:errorcluster)  [unwired: 2 in]
          }
        }
        n289 = property on="Camera Image Right" class="ImageControl"("Image Information Shown"=w437, "Image Information Visible"=w438) -> ()  [unwired: 2 in, 2 out]
        n290 = property on="Camera Image" class="ImageControl"("Image Information Shown"=w437, "Image Information Visible"=w438) -> ()  [unwired: 2 in, 2 out]
        n291 = call <vilib>:"WPI_DashboardNT Log FieldName Cache.vi"("Operation"=enum16{"Lookup/Add", "Index", "Clear"}."Clear") -> ()  [unwired: 8 in, 3 out]
      }
      event Panel Close {
        w460 = enum32{"Stop", "Record", "Playback"}."Stop" ("Rec Mode")
        # "Playback window has been closed, abort"
        n292 = event-data() -> ()  [unwired: 1 in, 4 out]
        n293 = local write "Rec Mode"(w460) -> ()
        n294 = global write "WPI_DashboardLogging Global.vi" "Recording"(w460) -> ()
      }
      event Panel Close {
        # "Abort playback window and ourself"
        n295 = event-data() -> ()  [unwired: 1 in, 4 out]
        n296 = invoke class="VI" method="FP.Close"(reference=w464) -> (reference out=w463:refnum<vi>)  [unwired: 2 in, 2 out]
        n297 = invoke class="VI" method="Abort VI"(reference=w463) -> (error out=w462:errorcluster)  [unwired: 2 in, 2 out]
        n298 = invoke class="VI" method="Abort VI"(error in=w462) -> ()  [unwired: 2 in, 3 out]
      }
      event User Event {
        n299 = event-data() -> ("IDs"=w471:cluster{"RPC field ID":u16, "Unique ID":u16}, "String"=w470:string)  [unwired: 1 in]
        n300 = Bundle("IDs"=w471, "String"=w470) -> (w469:T9)  [unwired: 1 in]
        n301 = call <vilib>:"Retrieve RPC Response.vi"("RPC Response"=w469) -> ("Output"=w467:string[][])  [unwired: 10 in]
        n302 = Build Array (concatenate)(w465, w467) -> (w466:string[][])
        n303 = local write "Command Params"(w466) -> ()
        n304 = local write "Cmd Status"("" ("Cmd Status")) -> ()
      }
      event "Tree": Double Click {
        n305 = event-data() -> ("PlatMods"=w477:T26, "Tag"=w474:string)  [unwired: 1 in]
        n306 = Unbundle(w477) -> ("Shift"=w476:bool)  [unwired: 4 out]
        n307 = String Subset(string=w474, length (rest)=1 ("length (rest)")) -> (substring=w473:string)  [unwired: 1 in]
        n308 = Not(x=w476) -> (.not. x?=w475:bool)
        n309 = case shown="\"/\"" w473 {
          tunnel: w474 -> [_ w480]
          tunnel: w475 -> [_ w479]
          frame Default {
          }
          frame "/" {
            n310 = call <vilib>:"NT Update Persistence.vi"("Persistence"=w479, "Name"=w480) -> ()  [unwired: 9 in, 1 out]
          }
        }
      }
    }
  }
  n311 = while {
    tunnel: w72 -> [w482]
    i -> [w485]
    stop <- FALSE stop-if-true
    n312 = Wait (ms)(milliseconds to wait=u32 100) -> ()  [unwired: 1 out]
    n313 = case shown="\"Playback\"" "Rec Mode" {
      tunnel: w485 -> [_ _ w500]
      tunnel: [u32 2829099 ("Base Color") u32 11141120 ("Target Color") w489] -> w481
      frame "Stop", Default {
        # "Reset the color, extra updates don't cost much"
      }
      frame "Record" {
      }
      frame "Playback" {
        # "Playback"
        n314 = Quotient & Remainder(x=w500, y=u32 50 ("milliseconds to wait")) -> (x-y*floor(x/y)=w496:u32)  [unwired: 1 out]
        n315 = Divide(x=w496, y=u32 50 ("milliseconds to wait")) -> (x/y=w493:dbl)
        n316 = Multiply(x=6.283185307179586, y=w493) -> (x*y=w498:dbl)
        n317 = Sine(x=w498) -> (sin(x)=w497:dbl)
        n318 = Absolute Value(x=w497) -> (abs(x)=w490:dbl)
        n319 = call "Interpolate RGB Color.vi"("Proportion"=w490, "Target Color"=u32 30976, "Base Color"=u32 2829099) -> ("Result Color"=w489:u32)  [unwired: 8 in]
      }
    }
    n320 = property class="Pane"(reference=w482, "PaneColor"=w481) -> ()  [unwired: 1 in, 2 out]
  }
  n321 = local write "Dashboard Tab"(T2."Drive" ("Dashboard Tab")) -> ()
  n322 = property on="On/Off" class="Bool (strict)"("Visible"=w43) -> ()  [unwired: 2 in, 2 out]
  n323 = property on="Motor" class="Clust (strict)"("Visible"=w43) -> ()  [unwired: 2 in, 2 out]
  n324 = property on="Progress" class="Clust (strict)"("Visible"=w43) -> ()  [unwired: 2 in, 2 out]
  n325 = property on="Test Ring" class="Ring (strict)"("Visible"=w43) -> ()  [unwired: 2 in, 2 out]
  n326 = call "IMAQ Create"("Image Name"="Image rotated", "Image Type"=w2) -> ("New Image"=w1:T5)  [unwired: 2 in, 2 out]
  n327 = property on="Rev/Fwd" class="Clust (strict)"("Visible"=w43) -> ()  [unwired: 2 in, 2 out]
  n328 = call "IMAQ Create"("Image Name"="Image Composite", "Image Type"=w8) -> ("New Image"=w4:T5)  [unwired: 2 in, 2 out]
  n329 = while {
    tunnel: u16 1741 ("timeout ms (25000)") -> [w502]
    stop <- FALSE stop-if-true
    n330 = TCP Create Listener(10:w502) -> (0:w501:errorcluster, 3:w503:refnum<k5>)  [unwired: 4 in, 1 out]
    n331 = case shown="No Error" w501 {
      selector: w501 -> [w505 _]
      tunnel: w503 -> [w506 _]
      frame No Error {
        n332 = while {
          tunnel: w506 -> [w509]
          tunnel: w505 -> [w508]
          stop <- FALSE stop-if-true
          n333 = TCP Wait On Listener(8:w508, 11:w509) -> (0:w510:errorcluster, 4:w511:refnum<k5>)  [unwired: 2 in, 3 out]
          n334 = local write "TCP"(w511) -> ()
          n335 = case shown="No Error" w510 {
            frame No Error {
            }
            frame Error {
              n336 = Wait (ms)(milliseconds to wait=u32 1000) -> ()  [unwired: 1 out]
            }
          }
        }
      }
      frame Error {
        n337 = Wait (ms)(milliseconds to wait=u32 1000) -> ()  [unwired: 1 out]
      }
    }
  }
  n338 = while {
    tunnel: w6 -> [w526]
    tunnel: w5 -> [w517]
    tunnel: w4 -> [w523]
    tunnel: w1 -> [w514]
    stop <- FALSE stop-if-true
    w515 = u32 2 items=["Horizontal", "Vertical", "Central", "1st Diagonal", "2nd Diagonal"] ("Type of Symmetry")
    n339 = call "IMAQ GetImageSize"("Image"=w526) -> ("Y Resolution"=w520:i32, "X Resolution"=w530:i32)  [unwired: 3 in, 1 out]
    n340 = call "IMAQ GetImageSize"("Image"=w517) -> ("Y Resolution"=w529:i32)  [unwired: 3 in, 2 out]
    n341 = Add(x=w520, y=w529) -> (x+y=w528:i32)
    n342 = call "IMAQ Symmetry"("Type of Symmetry"=w515, "Image Dst"=w514, "Image Src"=w517) -> ("Image Dst Out"=w516:T5)  [unwired: 2 in, 1 out]
    n343 = call "IMAQ SetImageSize"("Y Resolution"=w528, "X Resolution"=w530, "Image"=w523) -> ("Image Out"=w527:T5)  [unwired: 2 in, 1 out]
    n344 = Wait Until Next ms Multiple(millisecond multiple=u32 25) -> ()  [unwired: 1 out]
    n345 = Build Array(0, w520) -> (w521:i32[])
    n346 = call "IMAQ ImageToImage 2"("Image Src (Small)"=w526, "Image Src (Large)"=w527) -> ("error out"=w525:errorcluster, "Image Dst Out"=w524:T5)  [unwired: 8 in]
    n347 = call "IMAQ ImageToImage 2"("Offset Left/Top"=w521, "error in (no error)"=w525, "Image Src (Small)"=w516, "Image Src (Large)"=w524) -> ("Image Dst Out"=→"Camera Image":T5)  [unwired: 6 in, 1 out]
  }
  n348 = local write "Command Selection"(u16 0 ("milliseconds to wait")) -> ()
  n349 = local write "Command Params"(string[][] [] ("Command Params")) -> ()
  n350 = global write "WPI_DashboardLogging Global.vi" "Recording"(w66) -> ()
  n351 = local write "Rec Mode"(w66) -> ()
  n352 = call <vilib>:"NT Write String.vi"("String"="Select Auto", "Name"="Auto Selector") -> ()  [unwired: 9 in, 1 out]
